vi "בדיקת זמן ניתוק הממסר 6.vi"(7 "resultUserPrompt":bool, 8 "error":errorcluster, 11 "Path for Log":path) -> (0 "error out":errorcluster, 1 "בטוח כן/לא":bool, 2 "בדיקת זמן ניתוק הממסר":dbl)   [LabVIEW 2014]
uses:
  <instrlib>/niDMM/nidmm.llb/niDMM Function.ctl
  <instrlib>/niDMM/nidmm.llb/niDMM Resolution in Digits.ctl
  <vilib>/DAQmx/create/channels.llb/DAQmx Create Channel (DO-Digital Output).vi
  <vilib>/DAQmx/write.llb/DAQmx Write (Digital Bool 1Line 1Point).vi
  <instrlib>/niDMM/nidmm.llb/niDMM Configure Measurement Digits.vi
panel:
  # "Right-Click to\nexplain error"
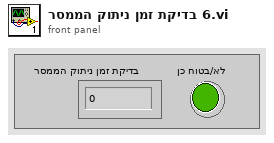
[diagram p1: front panel]
types:
  T1 = enum32{"Invalid", "Standard", "Closed", "Hidden", "Minimized", "Maximized"}
  T2 = typedef "niDMM Function.ctl" = enum16{"DC Volts", "AC Volts", "DC Current", "AC Current", "2-wire Resistance", "4-wire Resistance", "Diode", "Frequency", "Period", "AC Volts DC Coupled", "Capacitance", "Inductance", "Temperature"}
  T3 = typedef "niDMM Resolution in Digits.ctl" = dbl
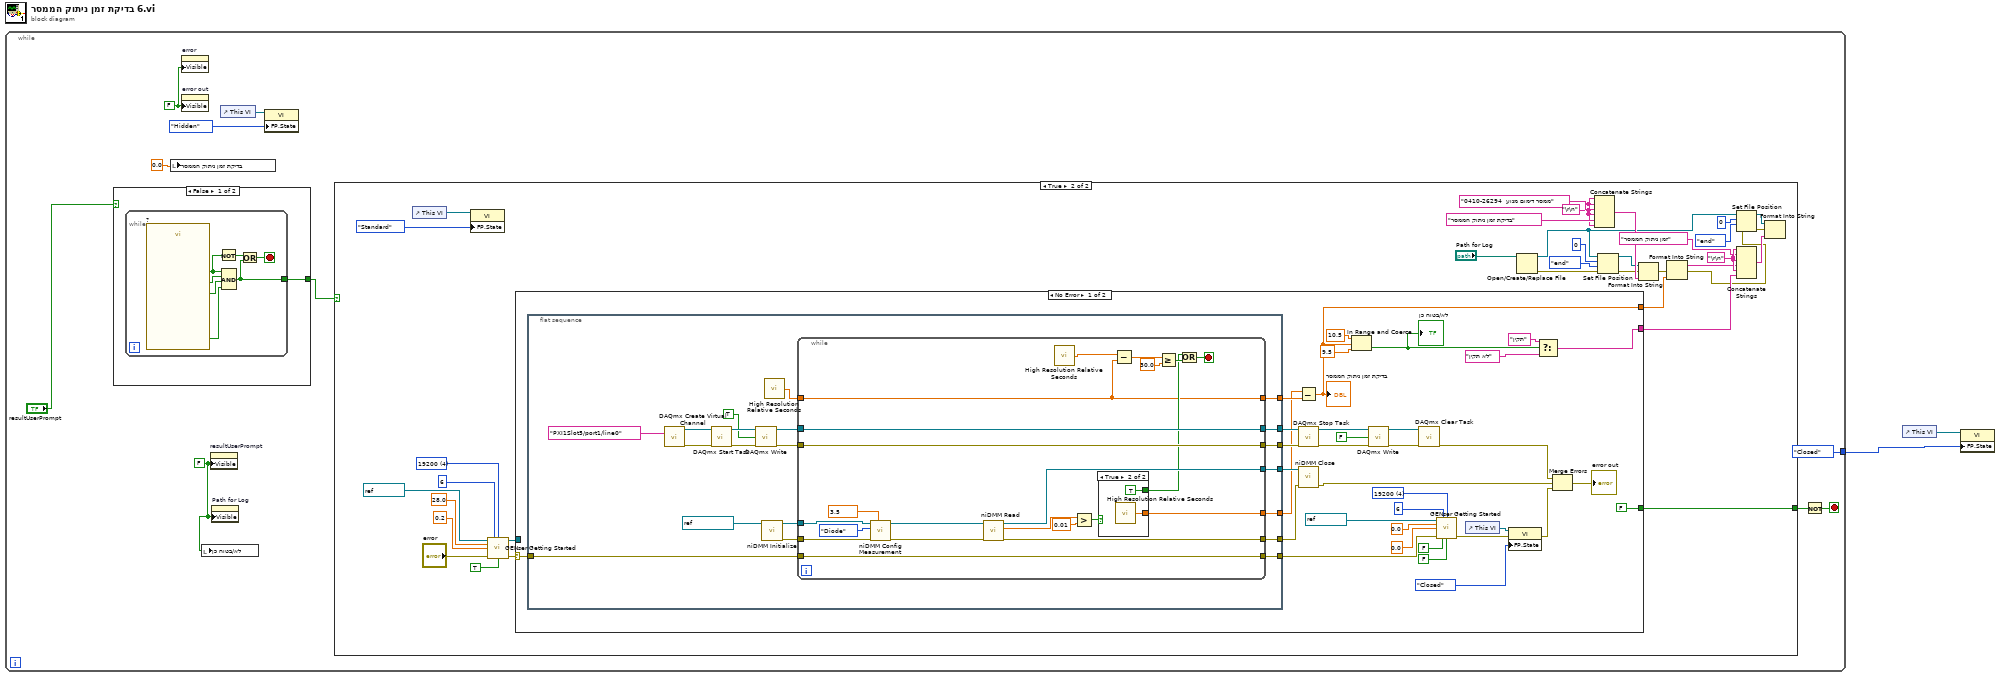
[diagram p0: block diagram]
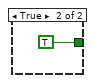
[diagram p2: hidden frame]
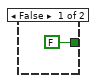
[diagram p3: hidden frame]
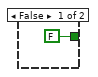
[diagram p4: hidden frame]
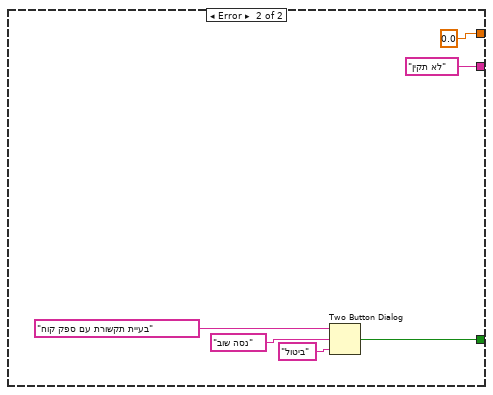
[diagram p5: hidden frame]
diagram:
  n1 = while {
    tunnel: [T1."Closed" ("Front Panel Window:State")] -> w1
    stop <- w11 stop-if-true
    w4 = FALSE ("Visible")
    w9 = FALSE ("Visible")
    n2 = case shown="False" "resultUserPrompt" {
      tunnel: [w13 TRUE] -> w12
      frame False {
        n3 = while {
          tunnel: [w14] -> w13
          stop <- w16 stop-if-true
          n4 = call "?"() -> ("הדקי הרב מודד"=w20:bool, "(מגע שלילי (מעטפת"=w19:bool, "C מגע חיובי"=w18:bool, "OK"=w15:bool)  [unwired: 15 in, 1 out]
          n5 = Not(x=w15) -> (.not. x?=w17:bool)
          n6 = Compound Arithmetic op=AND(w15, w18, w19, w20) -> (w14:bool)
          n7 = Or(x=w17, y=w14) -> (x .or. y?=w16:bool)
        }
      }
      frame True {
      }
    }
    n8 = local write "בדיקת זמן ניתוק הממסר"(0.0 ("זמן ניתוק הממסר")) -> ()
    n9 = property on="error" class="Clust (strict)"("Visible"=w9) -> ()  [unwired: 2 in, 2 out]
    n10 = property on="error out" class="Clust (strict)"("Visible"=w9) -> ()  [unwired: 2 in, 2 out]
    n11 = local write "בטוח כן/לא"(w4) -> ()
    n12 = property on="resultUserPrompt" class="Bool (strict)"("Visible"=w4) -> ()  [unwired: 2 in, 2 out]
    n13 = property on="Path for Log" class="Path"("Visible"=w4) -> ()  [unwired: 2 in, 2 out]
    n14 = control-ref of="This VI"() -> (w8:refnum<vi>)
    n15 = property class="VI"(reference=w8, "FP.State"=T1."Hidden" ("Front Panel Window:State")) -> ()  [unwired: 1 in, 2 out]
    n16 = case shown="True" w12 {
      tunnel: [FALSE ("T button?") w50] -> w10
      frame False {
      }
      frame True {
        w31 = "\r\n"
        w39 = "\r\n"
        w54 = u16 4 items=["1200", "2400", "4800", "9600", "19200"] ("BAUD")
        n17 = control-ref of="This VI"() -> (w49:refnum<vi>)
        n18 = property class="VI"(reference=w49, "FP.State"=T1."Standard" ("Front Panel Window:State")) -> ()  [unwired: 1 in, 2 out]
        n19 = call "GENser Getting Started.vi"("VISA"=refnum<visa-resource-name> "COM6", "GEN Addr"=i16 6, "BAUD"=w54, "Voltage Limit"=28.0, "Current Limit"=0.2, "error"="error", "Output On (T)"=TRUE) -> ("VISA out"=w55:refnum<visa-resource-name>, "error out"=w46:errorcluster)  [unwired: 5 in, 2 out]
        n20 = case shown="No Error" w46 {
          selector: w46 -> [w84 _]
          tunnel: w55 -> [_ _]
          tunnel: [FALSE ("T button?") w140] -> w50
          tunnel: [w62 0.0] -> w25
          tunnel: [w58 "לא תקין"] -> w24
          frame No Error {
            w79 = u16 4 items=["1200", "2400", "4800", "9600", "19200"] ("BAUD")
            n21 = flat-sequence {
              tunnel: [w106] -> w63
              tunnel: [w105] -> w64
              tunnel: [w104] -> w71
              tunnel: [w103] -> w72
              tunnel: [w102] -> w68
              tunnel: w84 -> [w101]
              tunnel: [w100] -> w83
              tunnel: [w99] -> w69
              frame #0 {
                n22 = call-poly <vilib>:"DAQmx Create Virtual Channel.vi"("lines"=tag "PXI1Slot5/port1/line0") -> ("task out"=w108:refnum<k21>, "error out"=w109:errorcluster)  [unwired: 13 in]
                n23 = call <vilib>:"DAQmx Start Task.vi"("task/channels in"=w108, "error in"=w109) -> ("task out"=w98:refnum<k21>, "error out"=w97:errorcluster)  [unwired: 12 in]
                n24 = call-poly <vilib>:"DAQmx Write.vi"("task/channels in"=w98, "data"=TRUE, "error in"=w97) -> ("task out"=w95:refnum<k21>, "error out"=w96:errorcluster)  [unwired: 10 in, 1 out]
                n25 = call <instrlib>:"niDMM Initialize.vi"("Instrument Descriptor"=refnum<k15> "PXI1Slot9") -> ("error out"=w110:errorcluster, "instrument handle out"=w111:refnum<k15>)  [unwired: 9 in]
                n26 = call <vilib>:"High Resolution Relative Seconds.vi"() -> ("relative seconds"=w93:dbl)
                n27 = while {
                  tunnel: [w114] -> w105
                  tunnel: [w132] -> w106
                  tunnel: [w125] -> w102
                  tunnel: [w117] -> w103
                  tunnel: [w116] -> w104
                  tunnel: [w124] -> w99
                  tunnel: w111 -> [w129]
                  tunnel: w110 -> [w128]
                  tunnel: w95 -> [w117]
                  tunnel: w96 -> [w116]
                  tunnel: [w118] -> w100
                  tunnel: w101 -> [w118]
                  tunnel: w93 -> [w114]
                  stop <- w121 stop-if-true
                  w134 = T3 3.5 items=["3 1/2"=3.5, "4 1/2"=4.5, "5 1/2"=5.5, "6 1/2"=6.5, "7 1/2"=7.5] ("Resolution in Digits")
                  n28 = call-poly <instrlib>:"niDMM Config Measurement.vi"("Resolution in Digits"=w134, "error in (no error)"=w128, "Function"=niDMM_Function."Diode", "instrument handle"=w129) -> ("error out"=w126:errorcluster, "instrument handle out"=w127:refnum<k15>)  [unwired: 6 in]
                  n29 = call <instrlib>:"niDMM Read.vi"("error in (no error)"=w126, "instrument handle"=w127) -> ("error out"=w124:errorcluster, "Measurement"=w131:dbl, "instrument handle out"=w125:refnum<k15>)  [unwired: 7 in]
                  n30 = call <vilib>:"High Resolution Relative Seconds.vi"() -> ("relative seconds"=w113:dbl)
                  n31 = Greater?(x=w131, y=0.01) -> (0:w119:bool)
                  n32 = case shown="True" w119 {
                    tunnel: [_ w137] -> w132
                    tunnel: [FALSE TRUE] -> w115
                    frame False {
                    }
                    frame True {
                      n33 = call <vilib>:"High Resolution Relative Seconds.vi"() -> ("relative seconds"=w137:dbl)
                    }
                  }
                  n34 = Subtract(x=w113, y=w114) -> (x-y=w123:dbl)
                  n35 = Greater Or Equal?(x=w123, y=30.0) -> (x >= y?=w120:bool)
                  n36 = Or(x=w115, y=w120) -> (x .or. y?=w121:bool)
                }
              }
            }
            n37 = Subtract(x=w63, y=w64) -> (x-y=w62:dbl)
            "בדיקת זמן ניתוק הממסר" <- w62
            n38 = call <vilib>:"DAQmx Stop Task.vi"("task/channels in"=w72, "error in"=w71) -> ("task out"=w77:refnum<k21>, "error out"=w76:errorcluster)  [unwired: 12 in]
            n39 = call <instrlib>:"niDMM Close.vi"("error in (no error)"=w69, "instrument handle"=w68) -> ("error out"=w67:errorcluster)  [unwired: 9 in]
            n40 = In Range and Coerce(upper limit=10.5, x=w62, lower limit=9.5) -> (In Range?=w59:bool)  [unwired: 1 out]
            "בטוח כן/לא" <- w59
            n41 = call-poly <vilib>:"DAQmx Write.vi"("task/channels in"=w77, "data"=FALSE, "error in"=w76) -> ("task out"=w74:refnum<k21>, "error out"=w75:errorcluster)  [unwired: 10 in, 1 out]
            n42 = call <vilib>:"DAQmx Clear Task.vi"("task in"=w74, "error in"=w75) -> ("error out"=w70:errorcluster)  [unwired: 13 in]
            n43 = call "GENser Getting Started.vi"("VISA"=refnum<visa-resource-name> "COM6", "GEN Addr"=i16 6, "BAUD"=w79, "Voltage Limit"=0.0, "Current Limit"=0.0, "error"=w83, "Reset (T)"=FALSE ("Output On (T)"), "Output On (T)"=FALSE) -> ("error out"=w85:errorcluster)  [unwired: 4 in, 3 out]
            n44 = control-ref of="This VI"() -> (w87:refnum<vi>)
            n45 = property class="VI"(reference=w87, error in=w85, "FP.State"=T1."Closed" ("Front Panel Window:State")) -> (error out=w81:errorcluster)  [unwired: 1 out]
            n46 = Select(t="תקין", s=w59, f="לא תקין") -> (s? t:f=w58:string)
            n47 = Merge Errors(w70, w67, w81) -> (→"error out":errorcluster)
          }
          frame Error {
            n48 = Two Button Dialog(message="בעיית תקשורת עם ספק קוח", 1:"ביטול" ("F button name (\"Cancel\")"), 2:"נסה שוב" ("T button name (\"OK\")")) -> (T button?=w140:bool)
          }
        }
        n49 = Open/Create/Replace File(file path (use dialog)="Path for Log") -> (refnum out=w26:refnum<file>, error out=w27:errorcluster)  [unwired: 5 in, 1 out]
        n50 = Concatenate Strings(w39, w39, "0410-26294  ממסר דימום מנוע", w39, "בדיקת זמן ניתוק הממסר", w39) -> (w43:string)
        n51 = Set File Position(offset (in bytes) (0)=i64 0, refnum=w26, from (0:start)=enum16{"start", "end", "current"}."end", error in=w27) -> (refnum out=w40:refnum<file>, error out=w38:errorcluster)
        n52 = Format Into String(initial string=w40, error in=w38, w43) -> (error out=w37:errorcluster)  [unwired: 1 in, 1 out]
        n53 = Format Into String(error in=w37, w25) -> (resulting string=w29:string, error out=w23:errorcluster)  [unwired: 2 in]
        n54 = Set File Position(offset (in bytes) (0)=i64 0, refnum=w26, from (0:start)=enum16{"start", "end", "current"}."end", error in=w23) -> (refnum out=w34:refnum<file>, error out=w35:errorcluster)
        n55 = Concatenate Strings(w31, "זמן ניתוק הממסר", w31, w29, w31, w24) -> (w36:string)
        n56 = Format Into String(initial string=w34, error in=w35, w36) -> ()  [unwired: 1 in, 2 out]
      }
    }
    n57 = Not(x=w10) -> (.not. x?=w11:bool)
  }
  n58 = control-ref of="This VI"() -> (w2:refnum<vi>)
  n59 = property class="VI"(reference=w2, "FP.State"=w1) -> ()  [unwired: 1 in, 2 out]
